vi "save active handles.vi"(8 "error in (no error)":errorcluster, 10 "Active Handles":variant[](array[variant]), 11 "Camera in":refnum<class "Camera.lvclass">) -> (0 "error out":errorcluster, 3 "Camera out":refnum<class "Camera.lvclass">)   [LabVIEW 2023, in "Camera.lvlib" / "Camera.lvclass"]
uses:
  Camera.lvclass
  Camera.lvclass/Camera.ctl
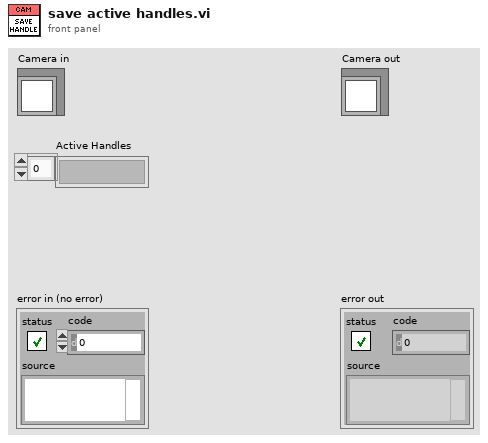
[diagram p1: front panel]
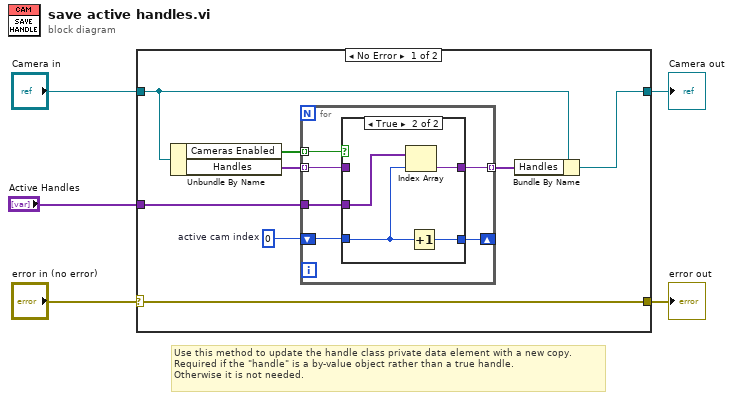
[diagram p0: block diagram]
diagram:
  # "Use this method to update the handle class private data element with a new copy.\nRequired if the \"handle\" is a by-value object rather than a true handle.\nOtherwise it is not needed."
  n1 = case shown="No Error" "error in (no error)" {
    selector: "error in (no error)" -> [w13 w27]
    tunnel: [w13 w27] -> w4
    tunnel: [w12 w26] -> w2
    tunnel: "Camera in" -> [w10 w26]
    tunnel: "Active Handles" -> [w11 _]
    frame No Error {
      w6 = 0  # active cam index
      n2 = Unbundle By Name(w10) -> ("Cameras Enabled"=w8:bool[], "Handles"=w9:variant[])
      n3 = for {
        tunnel: w11 -> [w17]
        tunnel: w9 -> [w18] mode=indexing
        tunnel: w8 -> [w19] mode=indexing
        tunnel: [w16] -> w7 mode=indexing
        shift-right: [w14] -> _
        shift-left: w6 -> [w15]
        n4 = case shown="True" w19 {
          tunnel: w18 -> [w21 _]
          tunnel: w17 -> [_ w25]
          tunnel: [w21 w24] -> w16
          tunnel: w15 -> [w20 w23]
          tunnel: [w20 w22] -> w14
          frame False {
          }
          frame True {
            n5 = Index Array(array=w25, index=w23) -> (element=w24:variant)
            n6 = Increment(x=w23) -> (x+1=w22:i32)
          }
        }
      }
      n7 = Bundle By Name(cluster=w10, "Handles"=w7) -> (w12:refnum<class "Camera.lvclass">)
    }
    frame Error {
    }
  }
  "error out" <- w4
  "Camera out" <- w2
